vi "ScpSetSampleFrequency.vi"(8 "error in (no error)":errorcluster, 10 "dSampleFrequency":dbl, 11 "hDevice in":u32) -> (0 "error out":errorcluster, 2 "dSampleFreqeuncySet":dbl, 3 "hDevice out":u32)   [LabVIEW 2018, in "LibTiePie.lvlib"]
uses:
  LibTiePie.lvlib
  LabViewHS4/libtiepie.dll
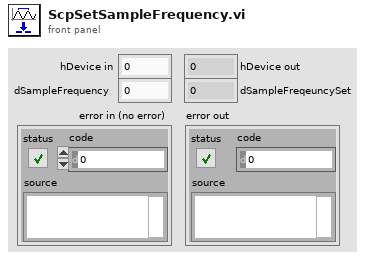
[diagram p1: front panel]
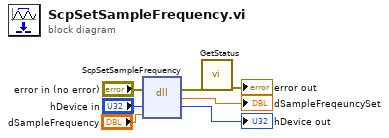
[diagram p0: block diagram]
diagram:
  n1 = dll-call lib="C:/Users/cwaha/Documents/LabViewHS4/libtiepie.dll" fn="ScpSetSampleFrequency"(error in="error in (no error)", "hDevice"="hDevice in", "dSampleFrequency"="dSampleFrequency") -> (error out=w7:errorcluster, "dSampleFreqeuncySet"=→"dSampleFreqeuncySet":dbl, "hDevice"=→"hDevice out":u32)  [unwired: 3 in, 1 out]
  n2 = call "GetStatus.vi"("error in (no error)"=w7) -> ("error out"=→"error out":errorcluster)  [unwired: 10 in]
